vi "Wait on Execution.vi"(8 "error in (no error)":errorcluster, 9 "Timeout mS (Forever)":i32=-1, 11 "Execution in":refnum<class "Execution.lvclass">) -> (0 "error out":errorcluster, 2 "Timeout?":bool, 3 "Execution out":refnum<class "Execution.lvclass">)   [LabVIEW 2020, in "TSnax.lvlib" / "Execution.lvclass"]
uses:
  Execution.lvclass
  Execution.lvclass/Execution.ctl
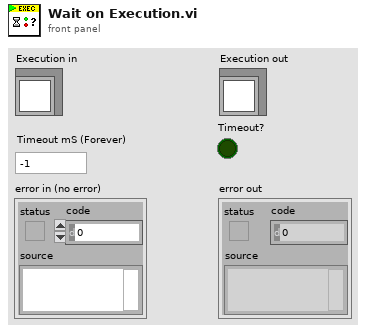
[diagram p1: front panel]
types:
  T1 = typedef "TSnax.lvlib/Execution.lvclass/Ref Data.ctl" = cluster{"Parameters":refnum<class "PropertyObject.lvclass">, "Client Sequence":refnum<class "SequenceFile.lvclass">, "Process Model":refnum<class "SequenceFile.lvclass">, "Entry Sequence":string, "Execution":refnum<k7>, "Report":refnum<class "Report.lvclass">, "Options":T2}
  T2 = typedef "TSnax.lvlib/Execution.lvclass/Execution Options.ctl" = cluster{"Use Default Model":bool, "Release Related References":bool}
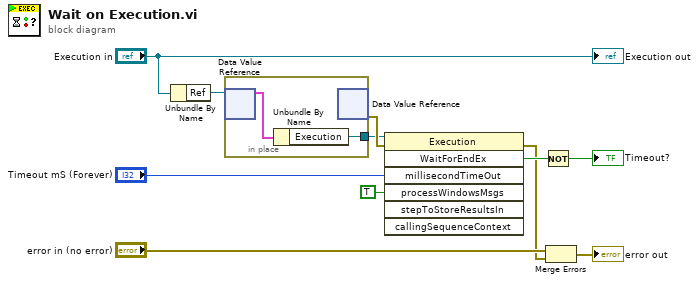
[diagram p0: block diagram]
diagram:
  n1 = Unbundle By Name("Execution in") -> ("Ref"=w9:refnum<data-value>)
  n2 = in-place {
    in-place-border: [w12] -> w7
    n3 = in-place-dvr #1(w9) -> (w13:T1)  [unwired: 1 out]
    n4 = Unbundle By Name(w13) -> ("Execution"=w12:refnum<k7>)
    n5 = in-place-dvr #1() -> (w11:errorcluster)  [unwired: 1 in, 1 out]
  }
  n6 = invoke class="Execution" method="WaitForEndEx"(reference=w7, error in=w11, "millisecondTimeOut"="Timeout mS (Forever)", "processWindowsMsgs"=TRUE) -> (error out=w1:errorcluster, "WaitForEndEx"=w4:bool)  [unwired: 3 in, 5 out]
  n7 = Not(x=w4) -> (.not. x?=→"Timeout?":bool)
  n8 = Merge Errors("error in (no error)", w1) -> (→"error out":errorcluster)
  "Execution out" <- "Execution in"
